vi "AcquireAndLog Loop.vi"(8 "error in (no error)":errorcluster, 9 "Message Queue":refnum<queue>, 10 "Acq and Log Queue":refnum<queue>, 11 "Acq and Logging Props":T1) -> ()   [LabVIEW 2013]
uses:
  Globals - Monitoring Variables.vi
  Globals - UI and RT Streams.vi
  Global - Configuration.vi
panel:
  in  "Log (current)\nFile Reference":refnum<k34>
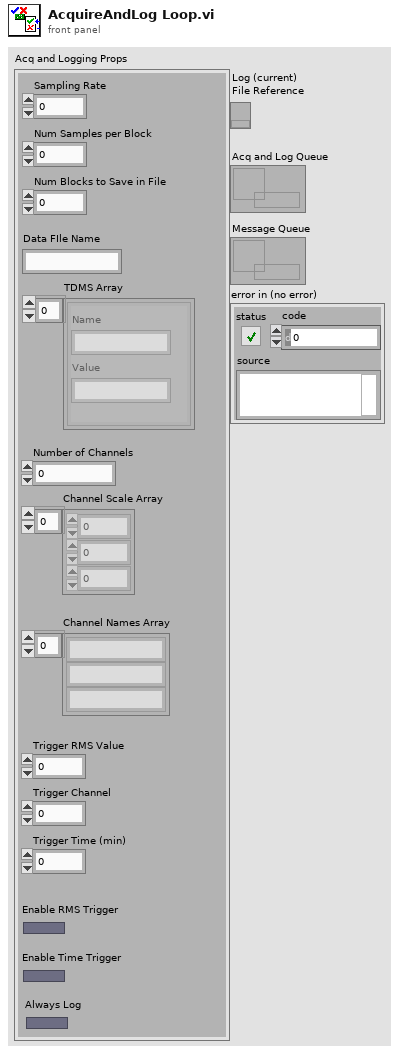
[diagram p1: front panel]
types:
  T1 = cluster{"Sampling Rate":dbl, "Num Samples per Block":i32, "Num Blocks to Save in File":i32, "Data FIle Name":string, "TDMS Array":cluster{"Name":string, "Value":string}[], "Number of Channels":i32, "Channel Scale Array":dbl[], "Channel Names Array":string[], "Trigger RMS Value":dbl, "Trigger Channel":i32, "Trigger Time (min)":i32, "Enable RMS Trigger":bool, "Enable Time Trigger":bool, "Always Log":bool}
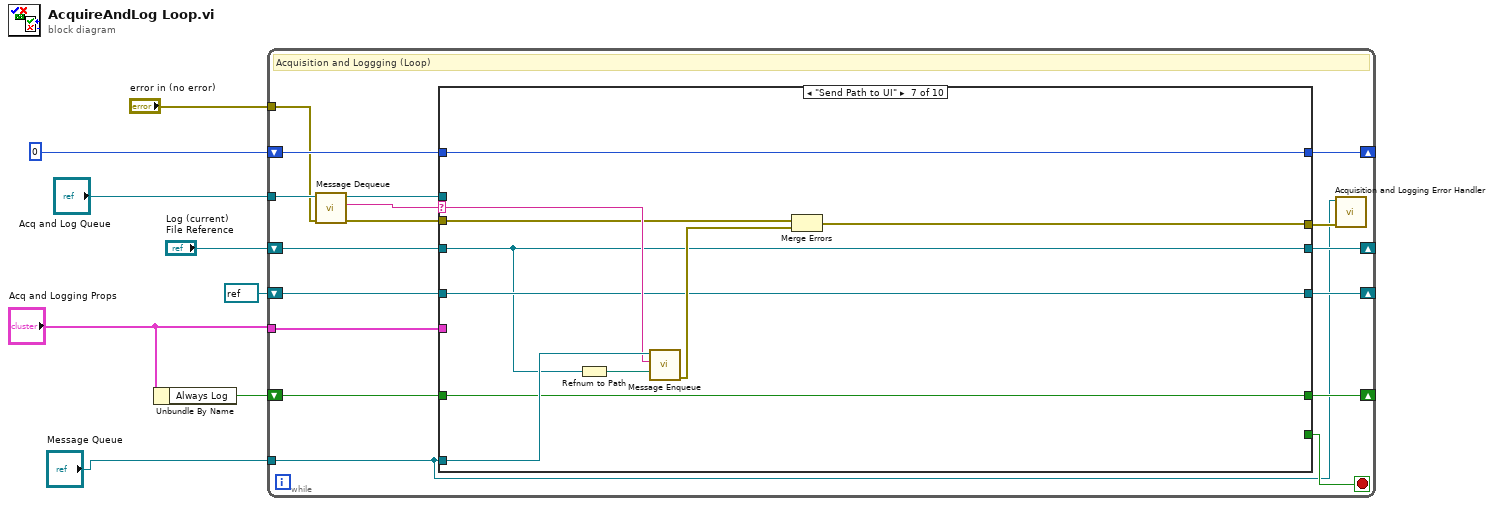
[diagram p0: block diagram]
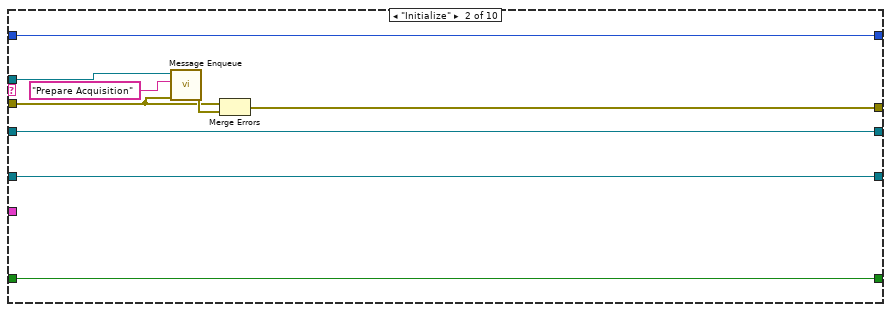
[diagram p3: hidden frame]
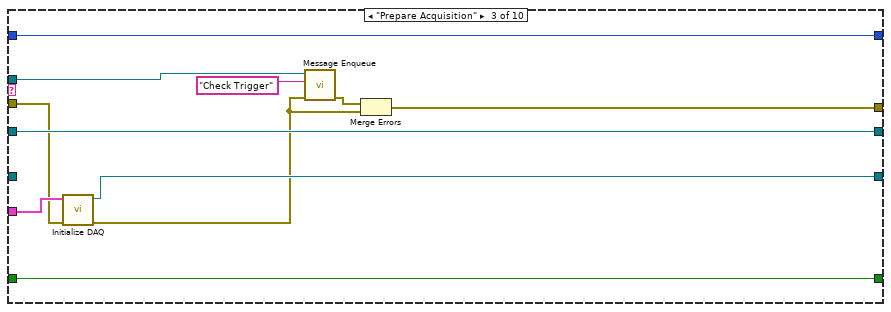
[diagram p4: hidden frame]
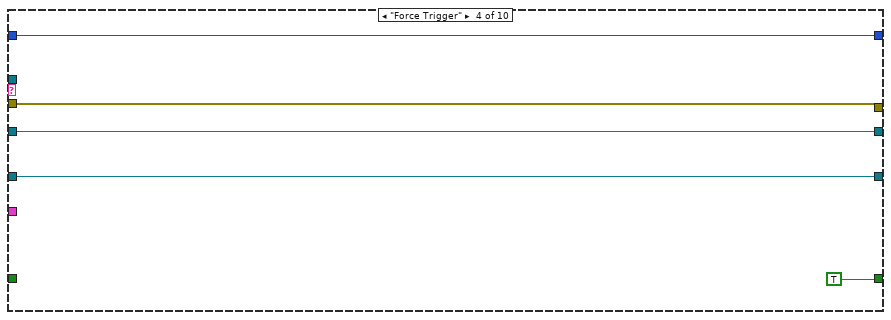
[diagram p5: hidden frame]
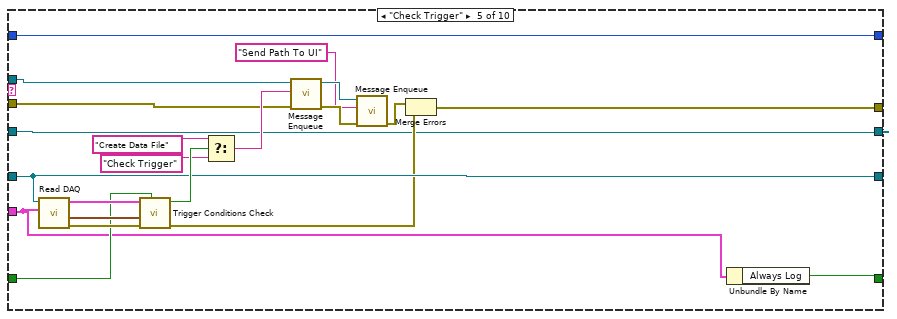
[diagram p6: hidden frame]
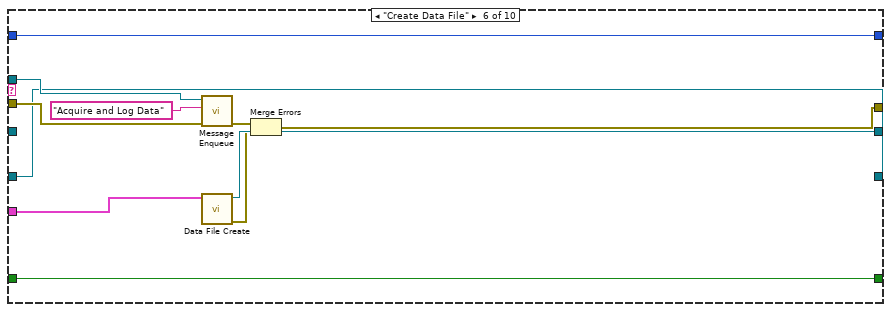
[diagram p7: hidden frame]
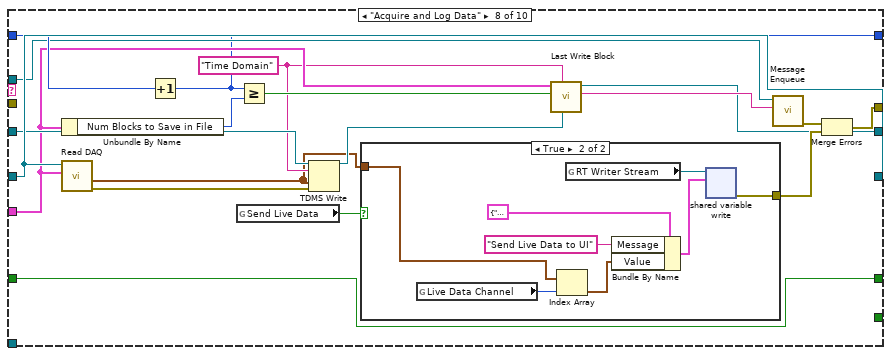
[diagram p8: hidden frame]
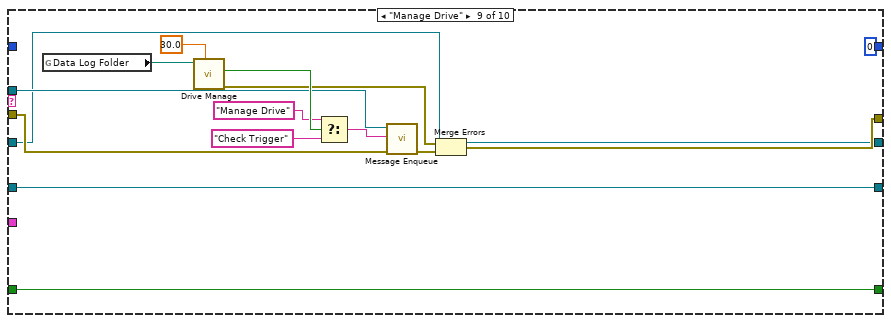
[diagram p10: hidden frame]
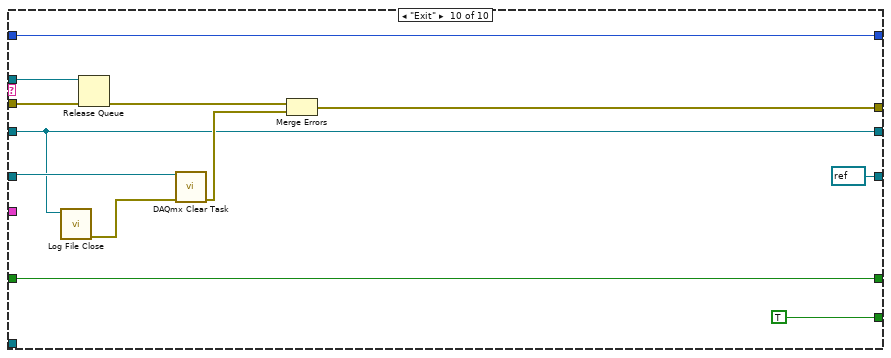
[diagram p11: hidden frame]
diagram:
  n1 = Unbundle By Name("Acq and Logging Props") -> ("Always Log"=w3:bool)
  n2 = while {
    tunnel: "Acq and Log Queue" -> [w24]
    tunnel: "Acq and Logging Props" -> [w21]
    shift-right: [w20] -> _
    shift-left: refnum<k21> refnum ("DAQmx Task Name") -> [w19]
    shift-right: [w18] -> _
    shift-left: "Log (current)\nFile Reference" -> [w17]
    shift-right: [w15] -> _
    shift-left: 0 -> [w16]
    shift-right: [w12] -> _
    shift-left: w3 -> [w13]
    tunnel: "Message Queue" -> [w10]
    tunnel: "error in (no error)" -> [w9]
    stop <- w14 stop-if-true
    # "Acquisition and Loggging (Loop)"
    n3 = call "Message Dequeue.vi"("error in (no error)"=w9, "Message Queue"=w24) -> ("error out"=w22:errorcluster, "Message"=w25:string, "Message Queue dup"=w23:refnum<queue>)  [unwired: 4 in, 1 out]
    n4 = case shown="\"Send Path to UI\"" w25 {
      selector: w25 -> [_ _ _ _ _ _ w95 _ _ _]
      tunnel: w23 -> [_ w39 w47 _ w73 w85 _ w109 w132 w148]
      tunnel: w22 -> [w27 w36 w41 w53 w67 w83 w93 _ w131 w147]
      tunnel: [w27 w35 w45 w53 w66 w82 w91 w100 w129 w143] -> w11
      tunnel: w21 -> [_ _ w49 _ w56 w77 _ w107 _ _]
      tunnel: [w28 w34 w48 w51 w68 w81 w90 w115 w125 refnum<k21> refnum ("DAQmx Task Name")] -> w20
      tunnel: w19 -> [w28 w34 _ w51 w68 w81 w90 w115 w125 w150]
      tunnel: [w29 w33 w44 w52 w59 w86 w89 w98 w126 w142] -> w18
      tunnel: w17 -> [w29 w33 w44 w52 w59 _ w89 w114 w126 w142]
      tunnel: w16 -> [w30 w32 w43 w54 w60 w78 w88 w112 _ w140]
      tunnel: [w30 w32 w43 w54 w60 w78 w88 w99 0 w140] -> w15
      tunnel: [_ _ _ _ _ _ _ _ _ TRUE] -> w14
      tunnel: w13 -> [w26 w31 w40 _ w57 w76 w87 w97 w124 w139]
      tunnel: w10 -> [_ _ _ _ _ _ w96 _ _ _]
      tunnel: [w26 w31 w40 TRUE w55 w76 w87 w97 w124 w139] -> w12
      frame "False", Default {
      }
      frame "Initialize" {
        n5 = call "Message Enqueue.vi"("error in (no error)"=w36, "Message"="Prepare Acquisition", "Message Queue"=w39) -> ("error out"=w37:errorcluster)  [unwired: 7 in, 1 out]
        n6 = Merge Errors(w36, w37) -> (w35:errorcluster)
      }
      frame "Prepare Acquisition" {
        n7 = call "Initialize DAQ.vi"("error in (no error)"=w41, "Acq and Logging Props"=w49) -> ("DAQmx Task Name"=w48:refnum<k21>)  [unwired: 8 in, 1 out]
        n8 = call "Message Enqueue.vi"("error in (no error)"=w41, "Message"="Check Trigger", "Message Queue"=w47) -> ("error out"=w42:errorcluster)  [unwired: 7 in, 1 out]
        n9 = Merge Errors(w42, w41) -> (w45:errorcluster)
      }
      frame "Force Trigger" {
      }
      frame "Check Trigger" {
        n10 = call "Read DAQ.vi"("Acq and Logging Props"=w56, "DAQmx Task Name"=w68) -> ("error out"=w74:errorcluster, "Waveform Data"=w75:waveform(dbl)[], "Acq and Logging Props dup"=w58:T1)  [unwired: 7 in]
        n11 = call "Trigger Conditions Check.vi"("Force Trigger?"=w57, "error in (no error)"=w74, "Waveform Data"=w75, "Acq and Logging Props"=w58) -> ("error out"=w65:errorcluster, "Trigger Condition Met?"=w72:bool)  [unwired: 6 in]
        n12 = Select(t="Create Data File", s=w72, f="Check Trigger") -> (s? t:f=w69:string)
        n13 = call "Message Enqueue.vi"("error in (no error)"=w67, "Message"=w69, "Message Queue"=w73) -> ("error out"=w63:errorcluster, "Message Queue dup"=w64:refnum<queue>)  [unwired: 7 in]
        n14 = call "Message Enqueue.vi"("error in (no error)"=w63, "Message"="Send Path To UI", "Message Queue"=w64) -> ("error out"=w61:errorcluster)  [unwired: 7 in, 1 out]
        n15 = Merge Errors(w61, w65) -> (w66:errorcluster)
        n16 = Unbundle By Name(w56) -> ("Always Log"=w55:bool)
      }
      frame "Create Data File" {
        n17 = call "Message Enqueue.vi"("error in (no error)"=w83, "Message"="Acquire and Log Data", "Message Queue"=w85) -> ("error out"=w80:errorcluster)  [unwired: 7 in, 1 out]
        n18 = call "Data File Create.vi"("Acq and Logging Props"=w77) -> ("error out"=w79:errorcluster, "TDMS File Reference"=w86:refnum<k34>)  [unwired: 9 in]
        n19 = Merge Errors(w80, w79) -> (w82:errorcluster)
      }
      frame "Send Path to UI" {
        n20 = Refnum to Path(1:w89) -> (0:w94:path)
        n21 = call "Message Enqueue.vi"("Value"=w94, "Message"=w95, "Message Queue"=w96) -> ("error out"=w92:errorcluster)  [unwired: 7 in, 1 out]
        n22 = Merge Errors(w93, w92) -> (w91:errorcluster)
      }
      frame "Acquire and Log Data" {
        w106 = "Time Domain" ("group name in (Untitled)")
        n23 = Unbundle By Name(w107) -> ("Num Blocks to Save in File"=w111:i32)
        n24 = call "Read DAQ.vi"("Acq and Logging Props"=w107, "DAQmx Task Name"=w115) -> ("error out"=w113:errorcluster, "Waveform Data"=w103:waveform(dbl)[])  [unwired: 7 in, 1 out]
        n25 = Increment(x=w112) -> (x+1=w99:i32)
        n26 = global read "Globals - Monitoring Variables.vi" "Send Live Data"() -> (w110:bool)
        n27 = Greater Or Equal?(x=w99, y=w111) -> (x >= y?=w108:bool)
        n28 = TDMS Write(0:w114, 5:w106, 9:w103, 11:w113) -> (4:w104:refnum<k34>)  [unwired: 2 in, 3 out]
        n29 = case shown="True" w110 {
          tunnel: w103 -> [_ w122]
          tunnel: [_ w116] -> w101
          frame False {
          }
          frame True {
            n30 = global read "Globals - Monitoring Variables.vi" "Live Data Channel"() -> (w123:u32)
            n31 = Index Array(array=w122, index=w123) -> (element=w120:waveform(dbl))
            n32 = global read "Globals - UI and RT Streams.vi" "RT Writer Stream"() -> (w117:refnum<k21>)
            n33 = Bundle By Name(cluster=cluster{"Message":string, "Value":variant} {"Message"="", "Value"=variant} ("Message Cluster"), "Message"="Send Live Data to UI", "Value"=w120) -> (w118:cluster{"Message":string, "Value":variant})
            n34 = shared-variable-write(w117, w118) -> (w116:errorcluster)  [unwired: 2 in, 2 out]
          }
        }
        n35 = call "Last Write Block.vi"("tdms file Ref"=w104, "Group Name TMDS"=w106, "End Block?"=w108, "Acq and Logging Props"=w107) -> ("Message"=w105:string, "tdms file out"=w98:refnum<k34>)  [unwired: 5 in, 1 out]
        n36 = call "Message Enqueue.vi"("Message"=w105, "Message Queue"=w109) -> ("error out"=w102:errorcluster)  [unwired: 8 in, 1 out]
        n37 = Merge Errors(w102, w101) -> (w100:errorcluster)
      }
      frame "Manage Drive" {
        n38 = global read "Global - Configuration.vi" "Data Log Folder"() -> (w138:path)
        n39 = call "Drive Manage.vi"("Min Drive Free Space (%)"=30.0, "Data Folder"=w138) -> ("error out"=w128:errorcluster, "Drive Space Below Limit"=w136:bool)  [unwired: 8 in]
        n40 = Select(t="Manage Drive", s=w136, f="Check Trigger") -> (s? t:f=w133:string)
        n41 = call "Message Enqueue.vi"("error in (no error)"=w131, "Message"=w133, "Message Queue"=w132) -> ("error out"=w127:errorcluster)  [unwired: 7 in, 1 out]
        n42 = Merge Errors(w128, w127) -> (w129:errorcluster)
      }
      frame "Exit" {
        n43 = call "Log File Close.vi"("Log File"=w142) -> ("error out"=w146:errorcluster)  [unwired: 10 in]
        n44 = Release Queue(queue=w148, error in (no error)=w147) -> (error out=w145:errorcluster)  [unwired: 1 in, 2 out]
        n45 = call <vilib>:"DAQmx Clear Task.vi"("task in"=w150, "error in"=w146) -> ("error out"=w144:errorcluster)  [unwired: 13 in]
        n46 = Merge Errors(w145, w144) -> (w143:errorcluster)
      }
    }
    n47 = call "Acquisition and Logging Error Handler.vi"("error in (no error)"=w11, "Message Queue"=w10) -> ()  [unwired: 9 in, 1 out]
  }
